vi "快速FFT变换.vi"() -> ()   [LabVIEW 2018]
uses:
  <vilib>/Analysis/2dsp.llb/Real FFT.vi
  <vilib>/Analysis/NI_AALBase.lvlib
  <vilib>/Analysis/NI_AALPro.lvlib
panel:
  out "相频曲线":dbl[](graph)
  out "幅频曲线":dbl[](graph)
  in  "停止":bool
  in  "噪声周期 2":dbl=1.0 caption="噪声周期2" format="%0.2f"
  in  "噪声幅值 2":dbl=1.0 caption="噪声幅值2" format="%0.2f"
  in  "噪声周期":dbl=1.0 format="%0.2f"
  in  "噪声幅值":dbl=1.0 format="%0.2f"
  out "时域波形":dbl[](graph)
  in  "周期":dbl=1.0 format="%0.2f"
  in  "幅值":dbl=1.0 format="%0.2f"
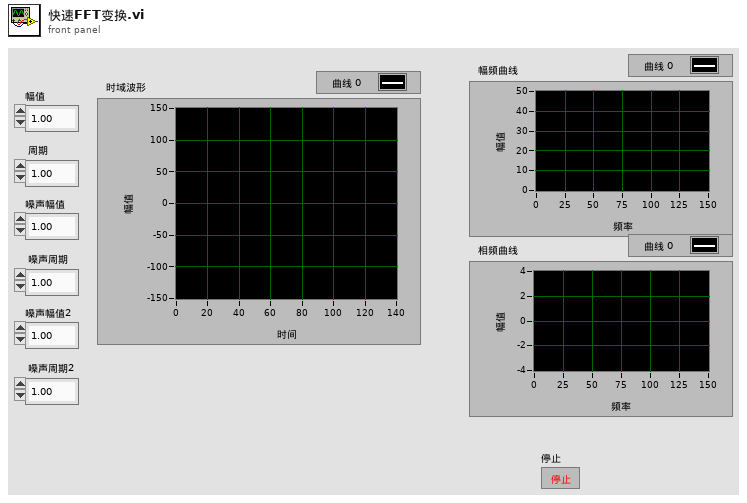
[diagram p1: front panel]
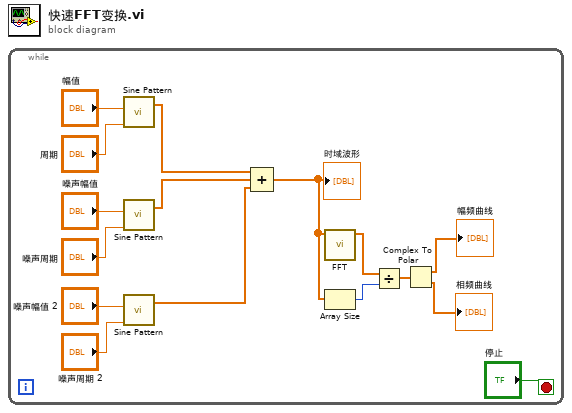
[diagram p0: block diagram]
diagram:
  n1 = while {
    stop <- "停止" stop-if-true
    n2 = call <vilib>:"Sine Pattern.vi"("cycles"="周期", "amplitude"="幅值") -> ("Sinusoidal Pattern"=w10:dbl[])  [unwired: 2 in, 1 out]
    n3 = call <vilib>:"Sine Pattern.vi"("cycles"="噪声周期", "amplitude"="噪声幅值") -> ("Sinusoidal Pattern"=w9:dbl[])  [unwired: 2 in, 1 out]
    n4 = call <vilib>:"Sine Pattern.vi"("cycles"="噪声周期 2", "amplitude"="噪声幅值 2") -> ("Sinusoidal Pattern"=w8:dbl[])  [unwired: 2 in, 1 out]
    n5 = Compound Arithmetic op=ADD(w10, w9, w8) -> (w4:dbl[])
    "时域波形" <- w4
    n6 = call-poly <vilib>:"FFT.vi"("X"=w4) -> ("FFT {X}"=w6:cdb[])  [unwired: 9 in, 1 out]
    n7 = Array Size(array=w4) -> (size(s)=w5:i32)
    n8 = Divide(x=w6, y=w5) -> (x/y=w3:cdb[])
    n9 = Complex To Polar(r * e^(i*theta)=w3) -> (r=→"幅频曲线":dbl[], theta=→"相频曲线":dbl[])
  }
